vi "Remove NaN.vi"(10 "Array in":dbl[][](array[numeric])) -> (2 "Array out":dbl[][](array[numeric]))   [LabVIEW 2019, in "Zen Analytics.lvlib" / "Zen Analytics.lvclass"]
uses:
  Zen Analytics.lvclass
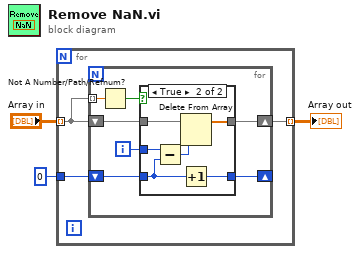
[diagram p0: block diagram]
diagram:
  n1 = for {
    tunnel: "Array in" -> [w6] mode=indexing
    tunnel: [w5] -> w2 mode=indexing
    tunnel: 0 ("length") -> [w4]
    n2 = for {
      tunnel: w6 -> [w13] mode=indexing
      shift-right: [w10] -> _
      shift-left: w4 -> [w11]
      shift-right: [w7] -> w5
      shift-left: w6 -> [w8]
      i -> [w9]
      n3 = Not A Number/Path/Refnum?(number/path/refnum=w13) -> (NaN/Path/Refnum?=w12:bool)
      n4 = case shown="True" w12 {
        tunnel: w8 -> [w14 w21]
        tunnel: w11 -> [w15 w16]
        tunnel: [w15 w19] -> w10
        tunnel: [w14 w20] -> w7
        tunnel: w9 -> [_ w17]
        frame False {
        }
        frame True {
          n5 = Subtract(x=w17, y=w16) -> (x-y=w18:i32)
          n6 = Delete From Array(array=w21, index=w18) -> (array with subset deleted=w20:dbl[])  [unwired: 1 in, 1 out]
          n7 = Increment(x=w16) -> (x+1=w19:i32)
        }
      }
    }
  }
  "Array out" <- w2
